vi "Is Cluster Terminal.vi"(10 "User VI Ref":refnum<vi>, 11 "Affected Items":T1) -> (1 "Data Type":variant, 2 "Refnum Term?":bool, 3 "Cluster Term?":bool)   [LabVIEW 2023]
doc: "Other parameter terminals other than those on a VI (checked in prior case). This will trurn true for VI cluster terminals, but we check this after, so this handles all others."
uses:
  top/BundleMagic.ctl
  <vilib>/Utility/Data Type/NI_Data Type.lvlib
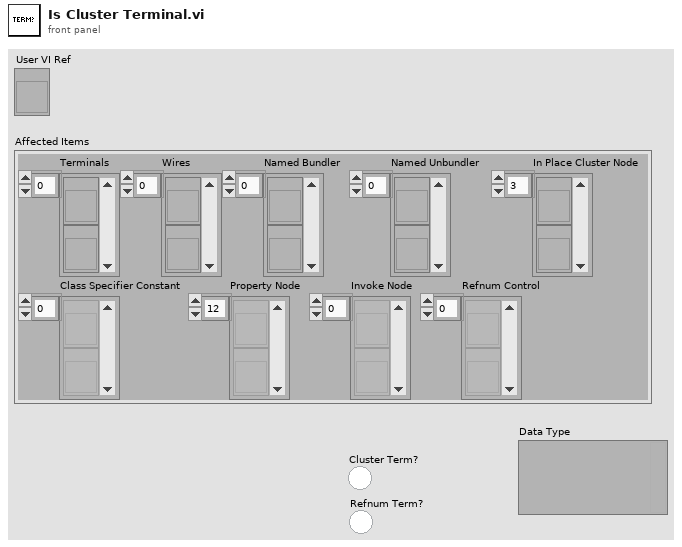
[diagram p1: front panel]
types:
  T1 = typedef "BundleMagic.ctl" = cluster{"Terminals":refnum<vi>[], "Wires":refnum<vi>[], "Named Bundler":refnum<vi>[], "Named Unbundler":refnum<vi>[], "In Place Cluster Node":refnum<vi>[], "Class Specifier Constant":refnum<vi>[], "Property Node":refnum<vi>[], "Invoke Node":refnum<vi>[], "Refnum Control":refnum<vi>[]}
  T2 = cluster{"Tunnel Ref":refnum<vi>, "On Tunnel?":bool, "Placement":enum32{"Choice 1", "Choice 2"}, "Tunnel Is Indexing?":bool, "Diagram":refnum<vi>, "Position":cluster{"Refnum":refnum<vi>, "Relative Direction":enum32{"Right", "Left", "Top", "Bottom", "Top Right", "Top Left", "Bottom Right", "Bottom Left"}, "Point32":cluster{"Horizontal":i32, "Vertical":i32}}, "Chosen Terminal":refnum<vi>, "Is Refnum?":bool, "Is Cluster?":bool, "Is Source?":bool, "Tunnel Direction":enum16{"In-Going", "Out-Going"}, "Tunnel Position":enum16{"Left", "Top", "Right", "Bottom"}, "Is Inner?":bool, "Terminal Is Indexing?":bool}
  T3 = typedef "NI_Data Type.lvlib/Data Type.ctl" = enum8{"Invalid Type", "Void", "I8", "I16", "I32", "I64", "U8", "U16", "U32", "U64", "Single Float", "Double Float", "Extended Float", "Single Complex", "Double Complex", "Extended Complex", "Enum U8", "Enum U16", "Enum U32", "Enum U64", "Single Float With Unit", "Double Float With Unit", "Extended Float With Unit", "Single Complex with Unit", "Double Complex with Unit", "Extended Complex with Unit", "Boolean", "String", "Path", "Picture", "Tag", "Array", "Cluster", "Variant", "LV Variant", "Waveform", "Timestamp", "Digital Waveform", "Digital Data", "ExpressData", "Refnum", "External Data", "VI", "Poly VI", "LabVIEW Class Instance", "Fixed Point", "Set Collection", "Map Collection"}
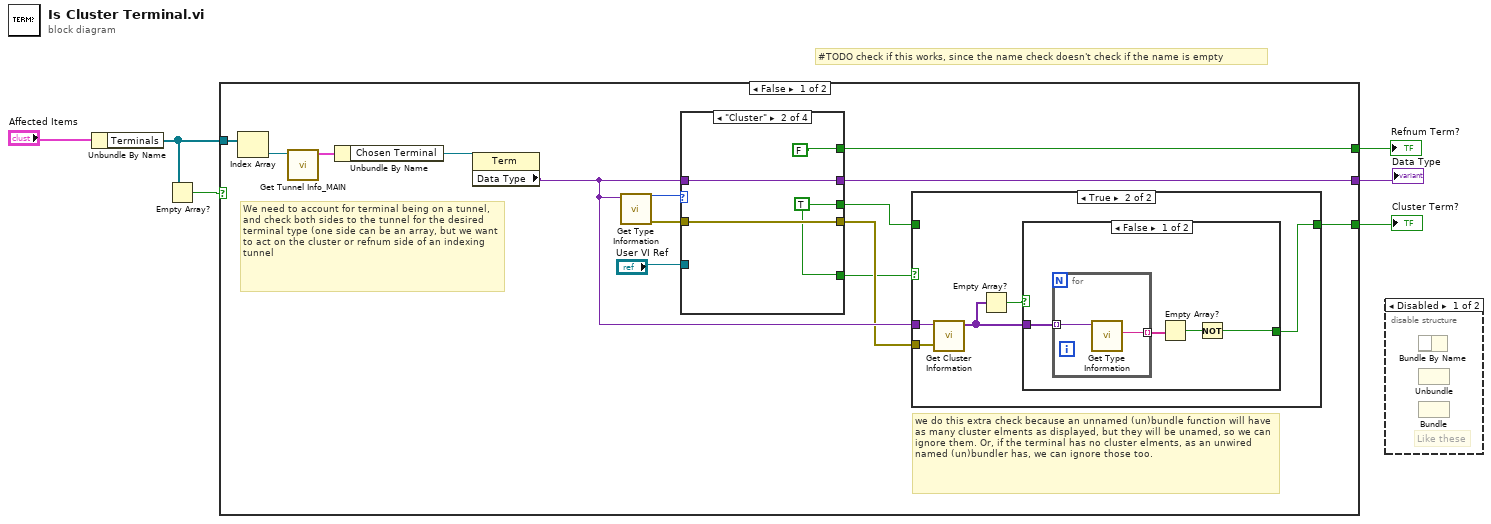
[diagram p0: block diagram]
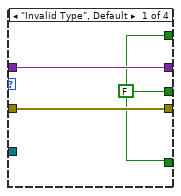
[diagram p2: hidden frame]
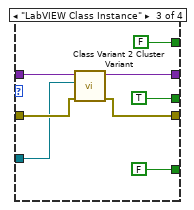
[diagram p3: hidden frame]
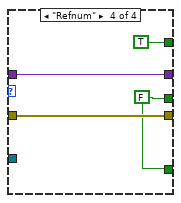
[diagram p4: hidden frame]
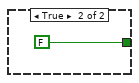
[diagram p6: hidden frame]
diagram:
  # "#TODO check if this works, since the name check doesn't check if the name is empty"
  n1 = Unbundle By Name("Affected Items") -> ("Terminals"=w3:refnum<vi>[])
  n2 = Empty Array?(array=w3) -> (empty?=w2:bool)
  n3 = case shown="False" w2 {
    tunnel: [w14 _] -> w5
    tunnel: [w17 _] -> w4
    tunnel: w3 -> [w16 _]
    tunnel: [w10 _] -> w1
    frame False {
      # "We need to account for terminal being on a tunnel, and check both sides to the tunnel for the desired terminal type (one side can be an array, but we want to act on the cluster or refnum side of an indexing tunnel"
      # "we do this extra check because an unnamed (un)bundle function will have as many cluster elments as displayed, but they will be unamed, so we can ignore them. Or, if the terminal has no cluster elments, as an unwired named (un)bundler has, we can ignore those too."
      n4 = Index Array(array=w16) -> (element=w8:refnum<vi>)  [unwired: 1 in]
      n5 = call "Get Tunnel Info_MAIN.vi"("Terminal in"=w8) -> ("Terminal Data Cluster"=w9:T2)  [unwired: 8 in, 2 out]
      n6 = Unbundle By Name(w9) -> ("Chosen Terminal"=w7:refnum<vi>)
      n7 = property class="Term"(reference=w7) -> ("Data Type"=w15:variant)  [unwired: 1 in, 2 out]
      n8 = call <vilib>:"Get Type Information.vi"("variant"=w15) -> ("error out"=w19:errorcluster, "type"=w20:T3)  [unwired: 6 in, 3 out]
      n9 = case shown="\"Cluster\"" w20 {
        tunnel: w15 -> [w22 w26 w35 w39]
        tunnel: [w23 w27 w33 w37] -> w13
        tunnel: w19 -> [w23 w27 w34 w37]
        tunnel: [w22 w26 w31 w39] -> w17
        tunnel: [w21 w25 TRUE w36] -> w12
        tunnel: "User VI Ref" -> [_ _ w30 _]
        tunnel: [w21 w25 FALSE w36] -> w11
        tunnel: [w21 FALSE FALSE TRUE] -> w10
        frame "Invalid Type", Default {
          w21 = FALSE
        }
        frame "Cluster" {
          w25 = TRUE
        }
        frame "LabVIEW Class Instance" {
          n10 = call "Class Variant 2 Cluster Variant.vi"("error in (no error)"=w34, "User VI Ref"=w30, "Variant"=w35) -> ("error out"=w33:errorcluster, "Control Value:Get"=w31:variant)  [unwired: 7 in]
        }
        frame "Refnum" {
          w36 = FALSE
        }
      }
      n11 = case shown="True" w11 {
        tunnel: w15 -> [_ w45]
        tunnel: [w40 w43] -> w14
        tunnel: w13 -> [_ w42]
        tunnel: w12 -> [w40 _]
        frame False {
          # "if invalid type, class, orrefnum, we won't do a check on its contents"
        }
        frame True {
          n12 = call <vilib>:"Get Cluster Information.vi"("error in (no error)"=w42, "variant"=w45) -> ("cluster elements"=w41:variant[])  [unwired: 8 in, 1 out]
          n13 = Empty Array?(array=w41) -> (empty?=w44:bool)
          n14 = case shown="False" w44 {
            tunnel: w41 -> [w49 _]
            tunnel: [w46 FALSE] -> w43
            frame False {
              n15 = for {
                tunnel: w49 -> [w51] mode=indexing
                tunnel: [w50] -> w48 mode=indexing
                n16 = call <vilib>:"Get Type Information.vi"("variant"=w51) -> ("name"=w50:string)  [unwired: 6 in, 4 out]
              }
              n17 = Empty Array?(array=w48) -> (empty?=w47:bool)
              n18 = Not(x=w47) -> (.not. x?=w46:bool)
            }
            frame True {
            }
          }
        }
      }
    }
    frame True {
    }
  }
  "Cluster Term?" <- w5
  "Data Type" <- w4
  "Refnum Term?" <- w1
  n19 = disable-structure shown="Disabled" {
    frame Disabled {
      # "Like these"
      n20 = Bundle By Name() -> ()  [unwired: 2 in, 1 out]
      n21 = Unbundle() -> ()  [unwired: 1 in, 2 out]
      n22 = Bundle() -> ()  [unwired: 3 in, 1 out]
    }
    frame Enabled {
    }
  }
